vi "Audio.vi"(7 "Delay_Enable":T1, 8 "index":i32, 10 "Delay_ticks":u32, 11 "Count(Ticks)":u32=907) -> (3 "Actual Period (tics)":u32)   [LabVIEW 2015]
uses:
  <vilib>/rvi/eio/common/nirviEmuTemplateMethod_errors.vi
  <vilib>/rvi/interface/RandomDataEmulation/niFpgaRandomDataHandleErrors.vi
  <vilib>/eio/EIONode/EIONode.xnode
  <vilib>/rvi/DataTransferAndStorage/Container/XNode/niFpgaContainer.xnode
  <vilib>/rvi/interface/RandomDataEmulation/nirviRandomDataFpgaReadWriteTemplate.vi
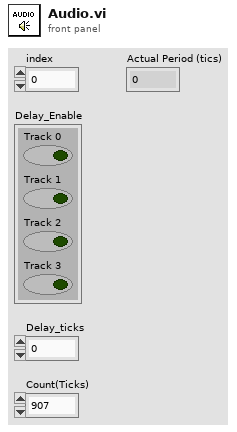
[diagram p1: front panel]
types:
  T1 = cluster{"Track 0":bool, "Track 1":bool, "Track 2":bool, "Track 3":bool}
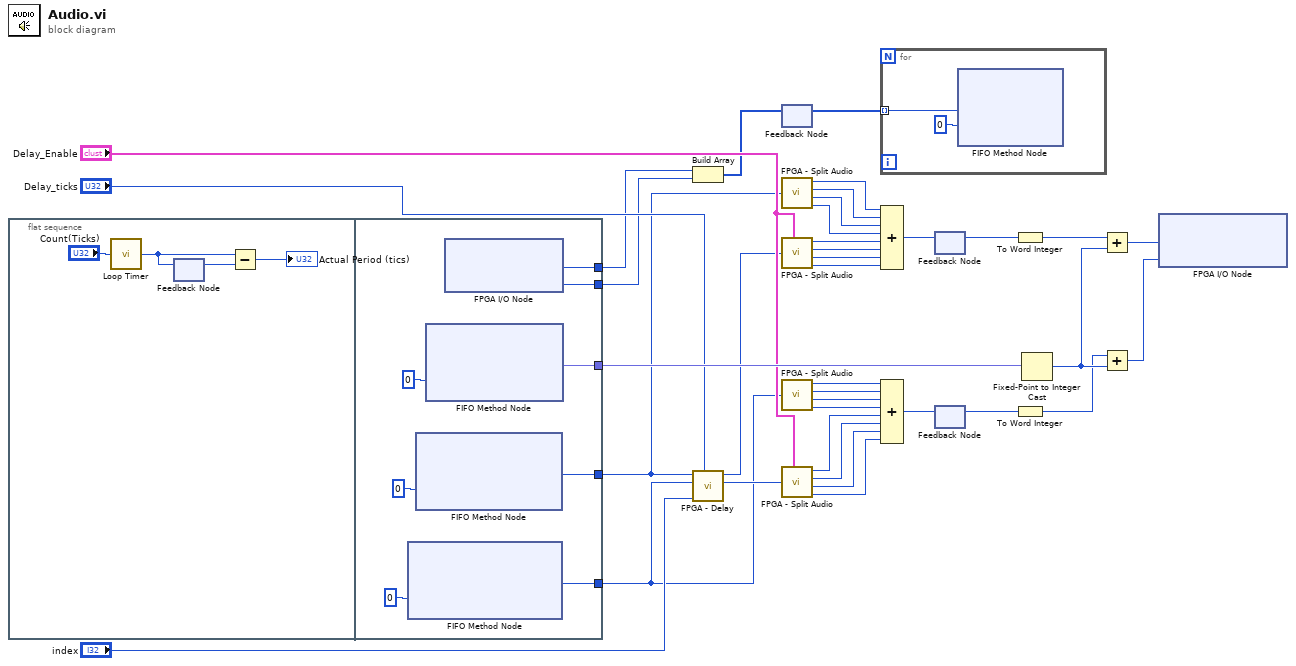
[diagram p0: block diagram]
diagram:
  n1 = flat-sequence {
    tunnel: [w49] -> w3
    tunnel: [w48] -> w13
    tunnel: [w47] -> w4
    tunnel: [w44] -> w15
    tunnel: [w42] -> w32
    frame #0 {
      n2 = call "Loop Timer"("Count(Ticks)"="Count(Ticks)") -> ("Tick Count(Ticks)"=w40:u32)
      n3 = feedback-in #1(w40) -> ()
      n4 = feedback #1() -> (w39:u32)  [unwired: 1 in]
      n5 = Subtract(x=w40, y=w39) -> (x-y=→"Actual Period (tics)":u32)
    }
    frame #1 {
      n6 = xnode ("FIFO Method Node")("Timeout"=0) -> ("Element"=w44:u64)  [unwired: 1 in, 2 out]
      n7 = xnode ("FIFO Method Node")("Timeout"=0) -> ("Element"=w48:u64)  [unwired: 1 in, 2 out]
      n8 = xnode ("FIFO Method Node")("Timeout"=0) -> ("Element"=w42:fxp<+/-,10,2>)  [unwired: 1 in, 2 out]
      n9 = xnode "FPGA I/O Node"() -> ("AudioIn/Left"=w49:i16, "AudioIn/Right"=w47:i16)  [unwired: 2 in, 2 out]
    }
  }
  n10 = Build Array(w3, w4) -> (w1:i16[])
  n11 = call "FPGA - Delay.vi"("Delay_ticks"="Delay_ticks", "index"="index", "Right Audio In"=w15, "Left Audio In"=w13) -> ("Delayed Right"=w20:u64, "Delayed Left"=w14:u64)  [unwired: 6 in]
  n12 = feedback #2() -> (w2:i16[])  [unwired: 1 in]
  n13 = feedback-in #2(w1) -> ()
  n14 = call "FPGA - Split Audio.vi"("U64 Audio In"=w13) -> ("Track 0 Out"=w5:u16, "Track 1 Out"=w6:u16, "Track 2 Out"=w7:u16, "Track 3 Out"=w8:u16)  [unwired: 4 in]
  n15 = call "FPGA - Split Audio.vi"("Enable"="Delay_Enable", "U64 Audio In"=w14) -> ("Track 0 Out"=w28:u16, "Track 1 Out"=w29:u16, "Track 2 Out"=w30:u16, "Track 3 Out"=w31:u16)  [unwired: 3 in]
  n16 = call "FPGA - Split Audio.vi"("U64 Audio In"=w15) -> ("Track 0 Out"=w16:u16, "Track 1 Out"=w17:u16, "Track 2 Out"=w18:u16, "Track 3 Out"=w19:u16)  [unwired: 4 in]
  n17 = call "FPGA - Split Audio.vi"("Enable"="Delay_Enable", "U64 Audio In"=w20) -> ("Track 0 Out"=w21:u16, "Track 1 Out"=w22:u16, "Track 2 Out"=w23:u16, "Track 3 Out"=w24:u16)  [unwired: 3 in]
  n18 = for {
    tunnel: w2 -> [w51] mode=indexing
    n19 = xnode ("FIFO Method Node")("Element"=w51, "Timeout"=0) -> ()  [unwired: 1 in, 2 out]
  }
  n20 = Compound Arithmetic op=ADD(w5, w6, w7, w8, w28, w29, w30, w31) -> (w9:u16)
  n21 = Compound Arithmetic op=ADD(w16, w17, w18, w19, w21, w22, w23, w24) -> (w11:u16)
  n22 = feedback #3() -> (w10:u16)  [unwired: 1 in]
  n23 = feedback-in #3(w9) -> ()
  n24 = feedback #4() -> (w12:u16)  [unwired: 1 in]
  n25 = feedback-in #4(w11) -> ()
  n26 = To Word Integer(number=w10) -> (16bit integer=w36:i16)
  n27 = To Word Integer(number=w12) -> (16bit integer=w33:i16)
  n28 = Fixed-Point to Integer Cast(1:w32) -> (0:w37:i16)
  n29 = Add(x=w36, y=w37) -> (x+y=w35:i16)
  n30 = Add(x=w33, y=w37) -> (x+y=w34:i16)
  n31 = xnode "FPGA I/O Node"("AudioOut/Left"=w35, "AudioOut/Right"=w34) -> ()  [unwired: 2 in, 2 out]
